vi "publisher tests Writer 10.vi"() -> ()   [LabVIEW 2018]
uses:
  publisher action.ctl
panel:
  out "Numeric":i32
  out "number":dbl
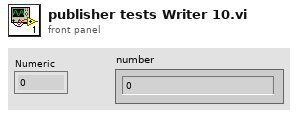
[diagram p1: front panel]
types:
  T1 = typedef "publisher action.ctl" = enum16{"set", "get", "init", "check"}
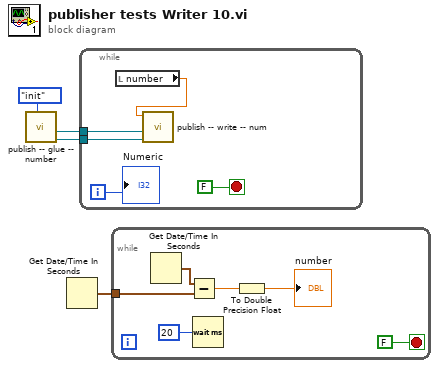
[diagram p0: block diagram]
diagram:
  n1 = call "publish -- glue -- number.vi"("publisher action"=publisher_action."init") -> ("request event"=w2:refnum<user-event>, "response out"=w1:refnum<user-event>)  [unwired: 8 in, 1 out]
  n2 = Get Date/Time In Seconds() -> (seconds since 1Jan1904=w4:timestamp)
  n3 = while {
    tunnel: w2 -> [w7]
    tunnel: w1 -> [w6]
    i -> [w8]
    stop <- FALSE stop-if-true
    n4 = local read "number"() -> (w5:dbl)
    n5 = call "publish -- write -- num.vi"("request event"=w7, "response in"=w6, "Numeric"=w5) -> ()  [unwired: 8 in, 1 out]
    "Numeric" <- w8
  }
  n6 = while {
    tunnel: w4 -> [w12]
    stop <- FALSE stop-if-true
    n7 = Get Date/Time In Seconds() -> (seconds since 1Jan1904=w14:timestamp)
    n8 = Subtract(x=w14, y=w12) -> (x-y=w15:dbl)
    n9 = Wait (ms)(milliseconds to wait=u32 20) -> ()  [unwired: 1 out]
    n10 = To Double Precision Float(number=w15) -> (double precision float=→"number":dbl)
  }
